vi "BotSpeak_Waitms.vi"(2 "Wait (ms)":dbl=1.0, 3 "Bot Settings":T1) -> (1 "Bot Settings 2":T1)   [LabVIEW 2012]
doc: "Causes VI to wait the specified number of milliseconds."
uses:
  <userlib>/BotSpeak/VIs/Direct/BotSpeak_Control.ctl
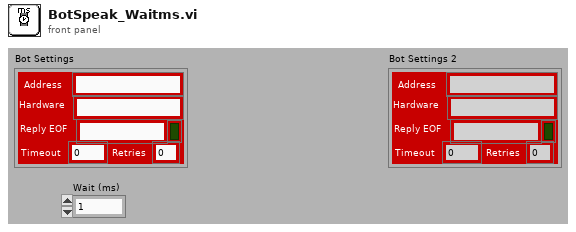
[diagram p1: front panel]
types:
  T1 = typedef "BotSpeak_Control.ctl" = cluster{"Address":string, "Reply EOF":string, "Hardware":string, "Retries":i8, "Timeout":i32, "Open?":bool}
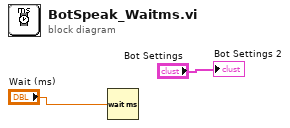
[diagram p0: block diagram]
diagram:
  n1 = Wait (ms)(milliseconds to wait="Wait (ms)") -> ()  [unwired: 1 out]
  "Bot Settings 2" <- "Bot Settings"
